vi "Redundant Micro.vi"(0 "GEA2 Reference In":refnum<k24>, 1 "GEA Inputs":T2 {"Destination" format="%.0x"; "Source" format="%.0x"}, 2 "Standalone?":bool, 11 "Error In":errorcluster) -> (4 "GEA2 Reference Out":refnum<k24>, 6 "Redundant Flood Condition":string, 8 "ERD Data Out":T1[](array[typedef]) {"ERD Number" format="%.0x"}, 10 "Redundant Pressure (inches)":dbl, 15 "Error Out":errorcluster)   [LabVIEW 2016, in "TL27.lvlib"]
doc: "This vi can be used to read ERD every 1 sec for user selected repeat counts."
uses:
  Projects/TL27.lvlib
  C:/Automation/DLLs/PC Dot Net/GeaCommunication.dll
  Common/LabVIEW GEA2 Toolkit/LabVIEW_GEA2_Toolkit.lvlibp/type defs/Source_Destination.ctl
  Common/LabVIEW GEA2 Toolkit/LabVIEW_GEA2_Toolkit.lvlibp/type defs/ERD Read Data Out.ctl
  Common/LabVIEW GEA2 Toolkit/LabVIEW_GEA2_Toolkit.lvlibp/type defs/ERD Read Data In.ctl
  Common/LabVIEW GEA2 Toolkit/LabVIEW_GEA2_Toolkit.lvlibp/type defs/Data Type.ctl
  Common/LabVIEW GEA2 Toolkit/LabVIEW_GEA2_Toolkit.lvlibp
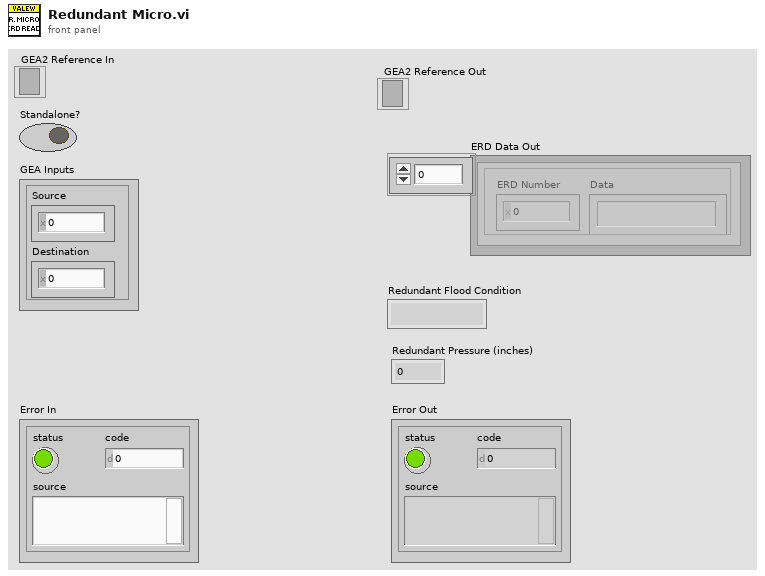
[diagram p1: front panel]
types:
  T1 = typedef "LabVIEW_GEA2_Toolkit.lvlibp/ERD Read Data Out.ctl" = cluster{"ERD Number":u16, "Data":string}
  T2 = typedef "LabVIEW_GEA2_Toolkit.lvlibp/Source_Destination.ctl" = cluster{"Source":u8, "Destination":u8}
  T3 = typedef "LabVIEW_GEA2_Toolkit.lvlibp/ERD Read Data In.ctl" = cluster{"ERD Number":u16, "Data Type":T4}
  T4 = typedef "LabVIEW_GEA2_Toolkit.lvlibp/Data Type.ctl" = enum16{"string", "boolean", "uint8_t", "uint16_t", "uint32_t", "uint64_t", "int8_t", "int16_t", "int32_t", "int64_t"}
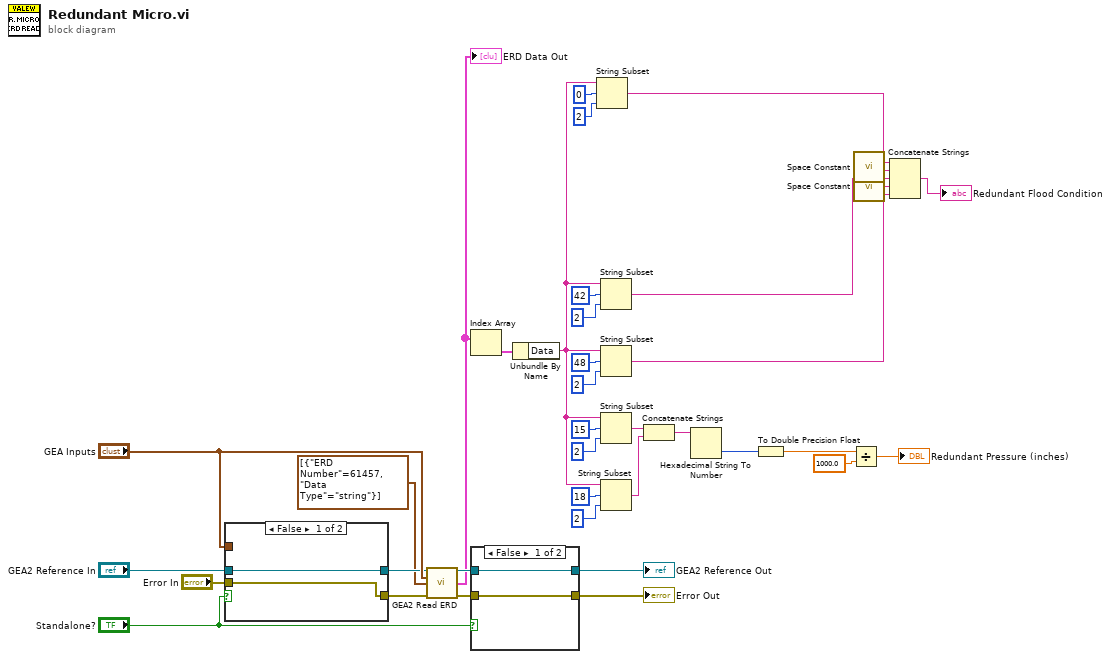
[diagram p0: block diagram]
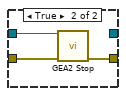
[diagram p2: hidden frame]
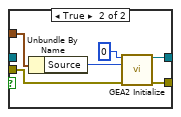
[diagram p3: hidden frame]
diagram:
  n1 = case shown="False" "Standalone?" {
    tunnel: "Error In" -> [w38 w45]
    tunnel: [w38 w44] -> w32
    tunnel: "GEA2 Reference In" -> [w39 _]
    tunnel: [w39 w43] -> w31
    tunnel: "GEA Inputs" -> [_ w41]
    frame False {
    }
    frame True {
      n2 = Unbundle By Name(w41) -> ("Source"=w42:u8)
      n3 = call "GEA2 Initialize.vi"("Board Index"=0, "Source Address"=w42, "error in"=w45) -> ("GEA2 Reference Out"=w43:refnum<k24>, "error out"=w44:errorcluster)  [unwired: 10 in, 1 out]
    }
  }
  n4 = call "GEA2 Read ERD.vi"("GEA2 Reference In"=w31, "GEA Inputs"="GEA Inputs", "Read ERD List"=T3[] [{"ERD Number"=61457, "Data Type"=enum."string"}], "Error In"=w32) -> ("GEA2 Reference Out"=w28:refnum<k24>, "ERD Data Out"=w11:T1[], "Error Out"=w29:errorcluster)  [unwired: 8 in, 1 out]
  "ERD Data Out" <- w11
  n5 = Index Array(array=w11) -> (element=w10:T1)  [unwired: 1 in]
  n6 = case shown="False" "Standalone?" {
    tunnel: w29 -> [w46 w49]
    tunnel: [w46 w48] -> w36
    tunnel: w28 -> [w47 w50]
    tunnel: [w47 _] -> w30
    frame False {
    }
    frame True {
      n7 = call "GEA2 Stop.vi"("GEA2 Reference In"=w50, "Error In"=w49) -> ("Error Out"=w48:errorcluster)  [unwired: 13 in]
    }
  }
  "Error Out" <- w36
  "GEA2 Reference Out" <- w30
  n8 = Unbundle By Name(w10) -> ("Data"=w9:string)
  n9 = String Subset(string=w9, offset (0)=0, length (rest)=2 ("length (rest)")) -> (substring=w7:string)
  n10 = String Subset(string=w9, offset (0)=42, length (rest)=2 ("length (rest)")) -> (substring=w1:string)
  n11 = String Subset(string=w9, offset (0)=48, length (rest)=2 ("length (rest)")) -> (substring=w2:string)
  n12 = String Subset(string=w9, offset (0)=15, length (rest)=2 ("length (rest)")) -> (substring=w21:string)
  n13 = String Subset(string=w9, offset (0)=18, length (rest)=2 ("length (rest)")) -> (substring=w20:string)
  n14 = Concatenate Strings(w21, w20) -> (w19:string)
  n15 = Hexadecimal String To Number(string=w19) -> (number=w18:u32)  [unwired: 2 in, 1 out]
  n16 = To Double Precision Float(number=w18) -> (double precision float=w13:dbl)
  n17 = Divide(x=w13, y=1000.0) -> (x/y=→"Redundant Pressure (inches)":dbl)
  n18 = call <vilib>:"Space Constant.vi"() -> ("String"=w4:string)
  n19 = call <vilib>:"Space Constant.vi"() -> ("String"=w3:string)
  n20 = Concatenate Strings(w7, w4, w1, w3, w2) -> (→"Redundant Flood Condition":string)
